vi "fileManipulation.vi"() -> ()   [LabVIEW 2025]
uses:
  <vilib>/numeric/Random Number (Range) DBL.vi
panel:
  out "Waveform Chart 2":dynamicdata(graph)
  in  "Path 2":path
  out "Waveform Chart":dbl(graph)
  out "temperature":dbl
  in  "write to file":bool
  in  "Path":path
  in  "lower limit":dbl
  in  "upper limit":dbl
  in  "?":bool
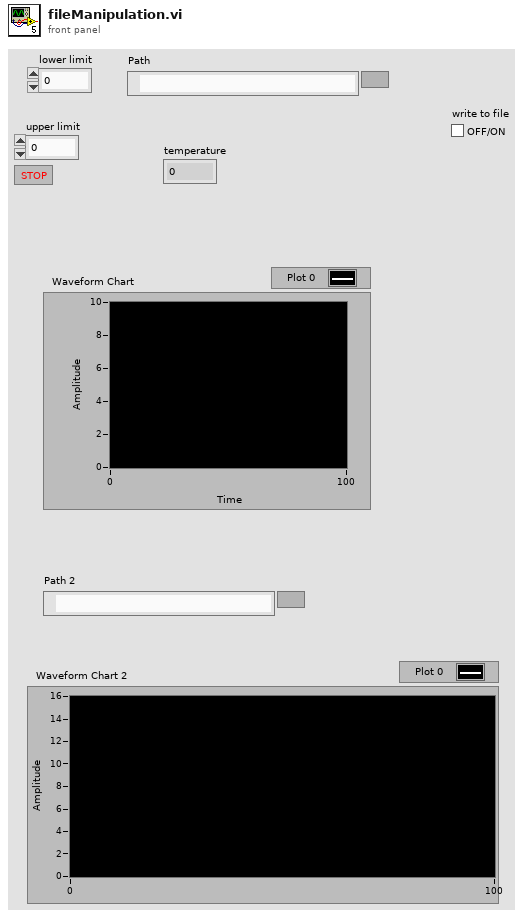
[diagram p1: front panel]
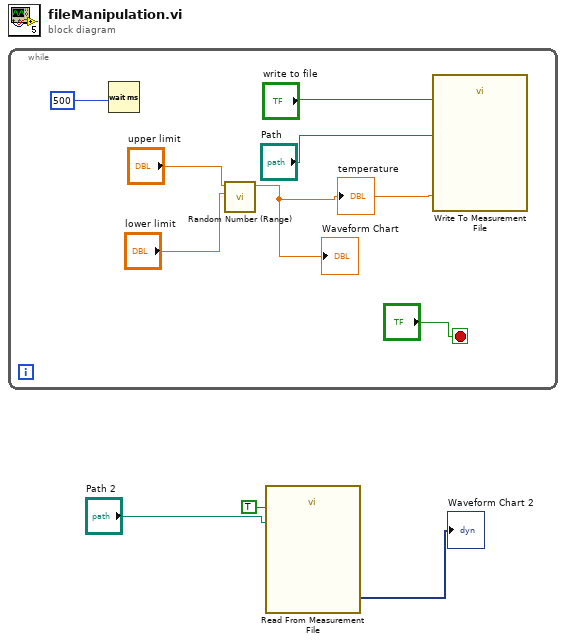
[diagram p0: block diagram]
diagram:
  n1 = while {
    stop <- "?" stop-if-true
    n2 = Wait (ms)(milliseconds to wait=u32 500 ("millisecond timer value")) -> ()  [unwired: 1 out]
    n3 = call-poly <vilib>:"Random Number (Range).vi"("lower bound (0)"="lower limit", "upper bound (100)"="upper limit") -> ("number"=w5:dbl)  [unwired: 9 in]
    "temperature" <- w5
    "Waveform Chart" <- w5
    n4 = call "Write To Measurement File"("Signals"=w5, "Enable"="write to file", "Filename"="Path") -> ()  [unwired: 14 in, 3 out]
  }
  n5 = call "Read From Measurement File"("Filename"="Path 2", "Enable"=TRUE) -> ("Signals"=→"Waveform Chart 2":dynamicdata)  [unwired: 4 in, 5 out]
